vi "parallax test.vi"() -> ()   [LabVIEW 2017]
uses:
  <vilib>/FPGAPlugInAG/myRIO-1900/niLvFpga_Open_myRIO-1900.vi
  <vilib>/rvi/interface/common/dynamic/niFpgaDynamicAddResources.vi
  <vilib>/Utility/error.llb/Error Cluster From Error Code.vi
  <vilib>/rvi/errors/niLvFpgaAdjustHostInterfaceError.vi
  <vilib>/rvi/interface/nirviOpenFPGA/nirviOpenFPGA.xnode
  myPAM_FPGATarget_FPGA(TopLevel-Pa_ueY72PW6EWo.lvbitx
  FPGA/FPGA (Top Level - Parallax).vi
  <vilib>/rvi/interface/nirviReadWriteControl/nirviReadWriteControl.xnode
  NiFpgaLv.dll
  <vilib>/rvi/interface/Simulation/niFpgaSimulationCallBeginRW.vi
panel:
  in  "toggle":bool
  in  "direction":enum16{"reverse", "stop", "forward"}(ring)
  in  "Stop Button":bool
  in  "input":dbl=60000.0
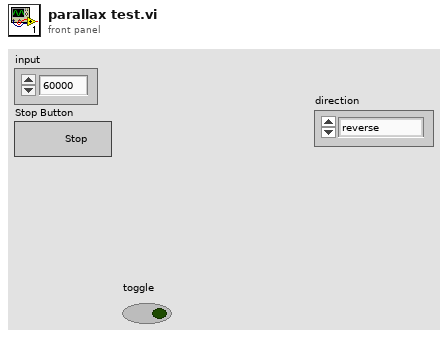
[diagram p1: front panel]
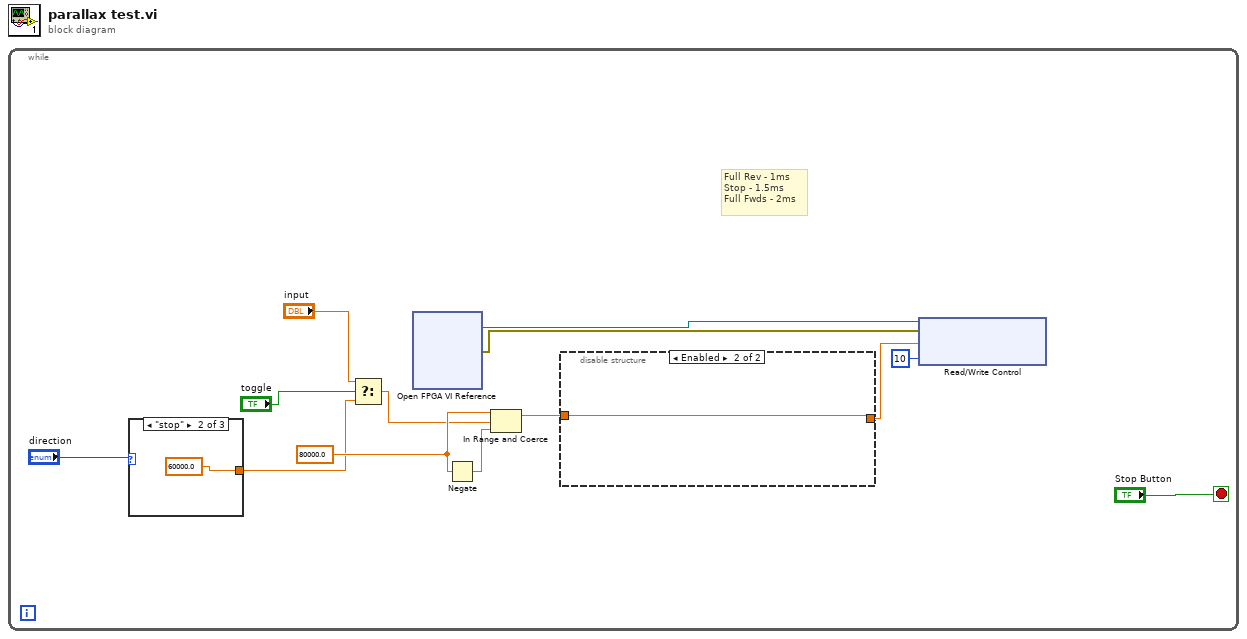
[diagram p0: block diagram]
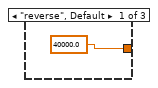
[diagram p2: hidden frame]
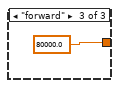
[diagram p3: hidden frame]
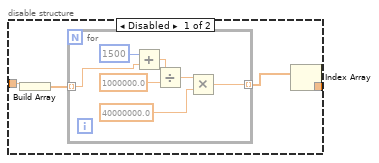
[diagram p4: hidden frame]
diagram:
  n1 = while {
    stop <- "Stop Button" stop-if-true
    w6 = 80000.0
    # "Full Rev - 1ms\nStop - 1.5ms\nFull Fwds - 2ms"
    n2 = case shown="\"stop\"" "direction" {
      tunnel: [40000.0 60000.0 80000.0] -> w3
      frame "reverse", Default {
      }
      frame "stop" {
      }
      frame "forward" {
      }
    }
    n3 = Select(t="input", s="toggle", f=w3) -> (s? t:f=w1:dbl)
    n4 = xnode "Open FPGA VI Reference"() -> ("FPGA VI Reference Out"=w13:refnum<k20>, "error out"=w12:errorcluster)  [unwired: 2 in]
    n5 = Negate(x=w6) -> (-x=w11:dbl)
    n6 = In Range and Coerce(upper limit=w6, x=w1, lower limit=w11) -> (coerced(x)=w8:dbl)  [unwired: 1 out]
    n7 = disable-structure shown="Enabled" {
      disable-tunnel: w8 -> [w20 w28]
      disable-tunnel: [w17 w28] -> w7
      frame Disabled {
        n8 = Build Array(w20) -> (w19:dbl[])
        n9 = for {
          tunnel: [w27] -> w18 mode=indexing
          tunnel: w19 -> [w21] mode=indexing
          n10 = Add(x=i16 1500 ("y"), y=w21) -> (x+y=w22:dbl)
          n11 = Divide(x=w22, y=1000000.0) -> (x/y=w25:dbl)
          n12 = Multiply(x=w25, y=40000000.0) -> (x*y=w27:dbl)
        }
        n13 = Index Array(array=w18) -> (element=w17:dbl)  [unwired: 1 in]
      }
      frame Enabled {
      }
    }
    n14 = xnode "Read/Write Control"("FPGA VI Reference In"=w13, "error in"=w12, "Pulse 2 Period (ticks)"=w7, "Pulse 1 Wait (ms)"=u16 10) -> ()  [unwired: 2 out]
  }
